vi "oax_Save Analog Tacho and Vibration Data.vi"(5 "reset? (F)":bool, 6 "channel name":string[](array[string]), 7 "tacho info":T1 {"slope (Rising)" items=["Rising", "Falling"]}, 8 "error in (no error)":errorcluster, 9 "channel info":T2[](array[typedef]) {"pregain" format="%.2f"; "weighting filter" items=["Linear", "A-weighting", "B-weighting", "C-weighting", "ITU-R 468-4", "Dolby", "CCITT", "C-message", "Wb", "Wc", "Wd", "We", "Wf", "Wh", "Wj", "Wk", "Wm", "AES17 20 kHz lowpass", "AES17 40 kHz lowpass", "AES17 20 kHz highpass", "AES17 40 kHz highpass"]; "dB reference" format="%^.1e"; "engineering units" items=["custom..."=0, "V"=1, "A"=21, "C"=30, "pC"=31, "s"=32, "-"=29, "Pa"=2, "N"=20, "g"=3, "m/s^2"=4, "m/s"=5, "m"=6, "mm/s"=12, "mm"=13, "micron/s"=14, "micron"=15, "in/s^2"=7, "in/s"=8, "in"=9, "mil/s"=10, "mil"=11, "rad/s^2"=16, "rad/s"=17, "rad"=18, "deg/s^2"=26, "deg/s"=27, "deg"=28, "RPM"=22, "cycle/s^2"=23, "Hz"=24, "cycle"=25, "strain"=19]; "sensor sensitivity" format="%#_5f"}, 10 "waveform data":waveform(dbl)[](array[waveform]), 11 "refnum":refnum<file>) -> (0 "error out":errorcluster, 3 "refnum out":refnum<file>)   [LabVIEW 2017]
doc: "Logs the tachometer and vibration data to a .dat file."
uses:
  <vilib>/addons/_NISVFA/_Shared subVIs/Controls/svc_Channel Info.ctl
  <vilib>/addons/_NISVFA/_Shared subVIs/Controls/svc_Engineering Units Text Ring.ctl
  <vilib>/addons/_NISVFA/_Shared subVIs/Controls/svc_Weighting Filter Text Ring.ctl
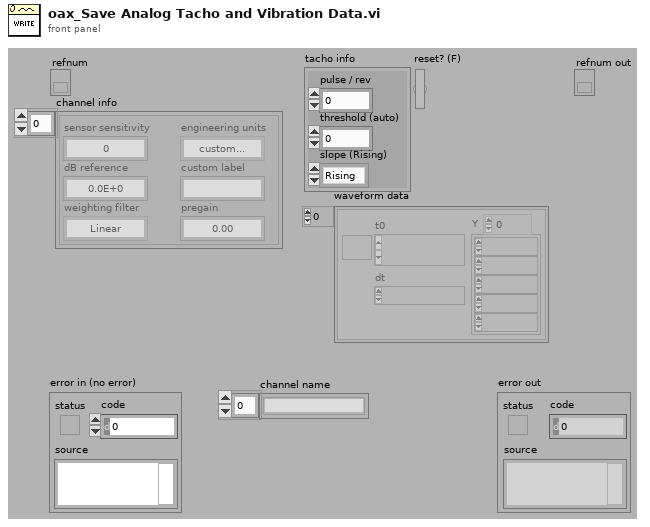
[diagram p1: front panel]
types:
  T1 = cluster{"pulse / rev":i32, "threshold (auto)":dbl, "slope (Rising)":u16}
  T2 = typedef "svc_Channel Info.ctl" = cluster{"sensor sensitivity":dbl, "engineering units":T3, "dB reference":dbl, "custom label":string, "weighting filter":T4, "pregain":dbl}
  T3 = typedef "svc_Engineering Units Text Ring.ctl" = u16
  T4 = typedef "svc_Weighting Filter Text Ring.ctl" = u16
  T5 = cluster{"pulse / rev":i32, "threshold (auto)":dbl, "slope (Rise)":enum16{"Rise", "Fall"}}
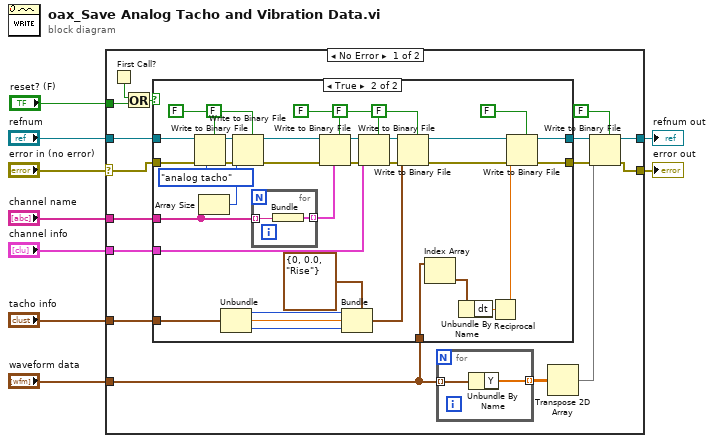
[diagram p0: block diagram]
diagram:
  n1 = case shown="No Error" "error in (no error)" {
    selector: "error in (no error)" -> [w24 w68]
    tunnel: [w18 w68] -> w8
    tunnel: "refnum" -> [w25 w67]
    tunnel: "channel name" -> [w23 _]
    tunnel: "channel info" -> [w22 _]
    tunnel: "tacho info" -> [w21 _]
    tunnel: "waveform data" -> [w15 _]
    tunnel: [w17 w67] -> w2
    tunnel: "reset? (F)" -> [w11 _]
    frame No Error {
      n2 = First Call?() -> (First Call?: T/F=w10:bool)
      n3 = Or(x=w10, y=w11) -> (x .or. y?=w12:bool)
      n4 = case shown="True" w12 {
        tunnel: w25 -> [w29 w64]
        tunnel: w24 -> [w28 w62]
        tunnel: w23 -> [_ w51]
        tunnel: w22 -> [_ w56]
        tunnel: w21 -> [_ w35]
        tunnel: [w28 w47] -> w19
        tunnel: [w29 w46] -> w20
        tunnel: w15 -> [_ w45]
        frame False {
        }
        frame True {
          n5 = Write to Binary File(file (use dialog)=w64, data=enum16{"analog tacho", "digital tacho"}."analog tacho", error in=w62, 5:FALSE ("prepend array or string size? (T)")) -> (refnum out=w60:refnum<file>, error out=w61:errorcluster)  [unwired: 2 in, 1 out]
          n6 = Array Size(array=w51) -> (size(s)=w59:i32)
          n7 = Unbundle(w35) -> ("pulse / rev"=w32:i32, "threshold (auto)"=w31:dbl, "slope (Rising)"=w30:u16)
          n8 = Write to Binary File(file (use dialog)=w60, data=w59, error in=w61, 5:FALSE ("prepend array or string size? (T)")) -> (refnum out=w52:refnum<file>, error out=w53:errorcluster)  [unwired: 2 in, 1 out]
          n9 = for {
            tunnel: w51 -> [w66] mode=indexing
            tunnel: [w65] -> w50 mode=indexing
            n10 = Bundle("ch0 string"=w66) -> (w65:cluster{"ch0 string":string})  [unwired: 1 in]
          }
          n11 = Write to Binary File(file (use dialog)=w52, data=w50, error in=w53, 5:FALSE ("prepend array or string size? (T)")) -> (refnum out=w54:refnum<file>, error out=w55:errorcluster)  [unwired: 2 in, 1 out]
          n12 = Bundle(cluster=T5 {"pulse / rev"=0, "threshold (auto)"=0.0, "slope (Rise)"=enum."Rise"} ("data"), "pulse / rev"=w32, "threshold (auto)"=w31, "slope (Rise)"=w30) -> (w33:T5)
          n13 = Write to Binary File(file (use dialog)=w54, data=w56, error in=w55, 5:FALSE ("prepend array or string size? (T)")) -> (refnum out=w57:refnum<file>, error out=w58:errorcluster)  [unwired: 2 in, 1 out]
          n14 = Write to Binary File(file (use dialog)=w57, data=w33, error in=w58, 5:FALSE ("prepend array or string size? (T)")) -> (refnum out=w48:refnum<file>, error out=w49:errorcluster)  [unwired: 2 in, 1 out]
          n15 = Index Array(array=w45) -> (element=w44:waveform(dbl))  [unwired: 1 in]
          n16 = Unbundle By Name(w44) -> ("dt"=w43:dbl)
          n17 = Reciprocal(x=w43) -> (1/x=w42:dbl)
          n18 = Write to Binary File(file (use dialog)=w48, data=w42, error in=w49, 5:FALSE ("prepend array or string size? (T)")) -> (refnum out=w46:refnum<file>, error out=w47:errorcluster)  [unwired: 2 in, 1 out]
        }
      }
      n19 = for {
        tunnel: w15 -> [w27] mode=indexing
        tunnel: [w26] -> w16 mode=indexing
        n20 = Unbundle By Name(w27) -> ("Y"=w26:dbl[])
      }
      n21 = Transpose 2D Array(2D array=w16) -> (transposed array=w14:dbl[][])
      n22 = Write to Binary File(file (use dialog)=w20, data=w14, error in=w19, 5:FALSE ("prepend array or string size? (T)")) -> (refnum out=w17:refnum<file>, error out=w18:errorcluster)  [unwired: 2 in, 1 out]
    }
    frame Error {
    }
  }
  "error out" <- w8
  "refnum out" <- w2
